vi "xijk_compensate_fwhm_gaussian.vi"(10 "FWHM":dbl) -> (2 "Numeric":dbl)   [LabVIEW 2009]
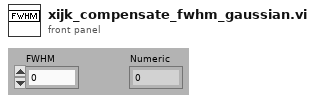
[diagram p1: front panel]
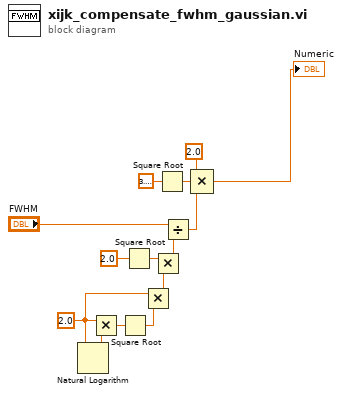
[diagram p0: block diagram]
diagram:
  w10 = 2.0 ("y")
  n1 = Natural Logarithm(1:w10) -> (0:w12:dbl)
  n2 = Multiply(x=w10, y=w12) -> (x*y=w11:dbl)
  n3 = Square Root(x=w11) -> (sqrt(x)=w9:dbl)
  n4 = Square Root(x=2.0 ("value")) -> (sqrt(x)=w5:dbl)
  n5 = Multiply(x=w10, y=w9) -> (x*y=w8:dbl)
  n6 = Multiply(x=w5, y=w8) -> (x*y=w6:dbl)
  n7 = Square Root(x=3.141592653589793) -> (sqrt(x)=w1:dbl)
  n8 = Divide(x="FWHM", y=w6) -> (x/y=w3:dbl)
  n9 = Compound Arithmetic op=MULTIPLY(2.0 ("value"), w1, w3) -> (→"Numeric":dbl)
